vi "LA_data_decode_Rev01.vi"(10 "Data In":u8[](array[numeric])) -> (0 "Bytes Received":dbl, 1 "Time stamp":dbl, 2 "Data Bytes":dbl, 3 "RG15":u8[](array[numeric]), 4 "RG14":u8[](array[numeric]), 5 "All data":u8[](array[numeric]))   [LabVIEW 2012]
panel:
  out "Numeric 4":dbl
  out "Numeric 3":dbl
  out "Numeric 2":dbl
  out "Numeric":dbl
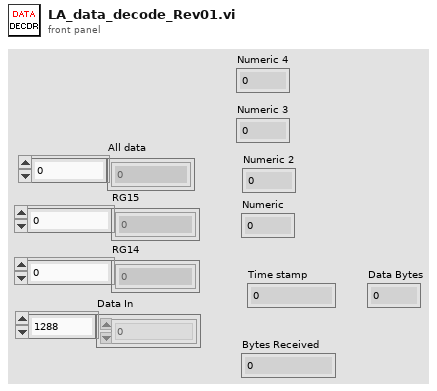
[diagram p1: front panel]
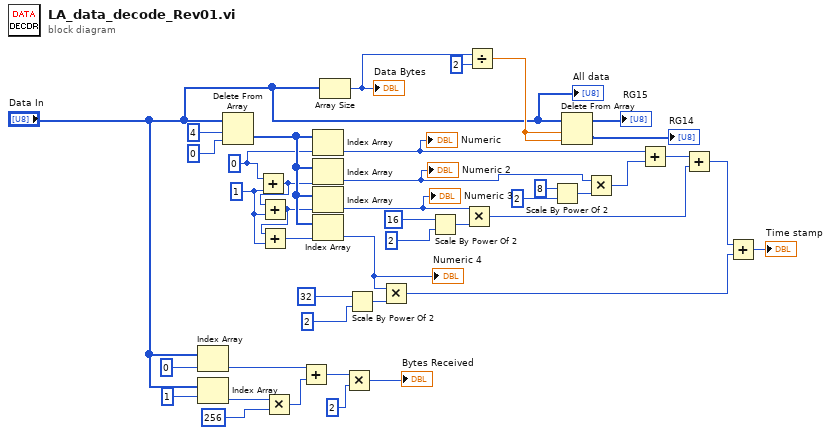
[diagram p0: block diagram]
diagram:
  w11 = 0
  w34 = 1
  n1 = Index Array(array="Data In", index=0) -> (element=w17:u8)
  n2 = Index Array(array="Data In", index=1) -> (element=w16:u8)
  n3 = Delete From Array(array="Data In", length=4, index=0) -> (deleted portion=w37:u8[])  [unwired: 1 out]
  n4 = Add(x=w11, y=w34) -> (x+y=w6:i32)
  n5 = Add(x=w6, y=w34) -> (x+y=w35:i32)
  n6 = Add(x=w35, y=w34) -> (x+y=w30:i32)
  n7 = Multiply(x=w16, y=256) -> (x*y=w39:i32)
  n8 = Add(x=w17, y=w39) -> (x+y=w10:i32)
  n9 = Index Array(array=w37, index=w11) -> (element=w15:u8)
  "Numeric" <- w15
  n10 = Index Array(array=w37, index=w6) -> (element=w14:u8)
  "Numeric 2" <- w14
  n11 = Index Array(array=w37, index=w35) -> (element=w13:u8)
  "Numeric 3" <- w13
  n12 = Index Array(array=w37, index=w30) -> (element=w12:u8)
  "Numeric 4" <- w12
  n13 = Array Size(array="Data In") -> (size(s)=w5:i32)
  "Data Bytes" <- w5
  n14 = Multiply(x=w10, y=2) -> (x*y=→"Bytes Received":i32)
  n15 = Scale By Power Of 2(n=32, x=2) -> (x*2^n=w33:i32)
  n16 = Multiply(x=w12, y=w33) -> (x*y=w19:i32)
  n17 = Scale By Power Of 2(n=16, x=2) -> (x*2^n=w29:i32)
  n18 = Multiply(x=w13, y=w29) -> (x*y=w21:i32)
  n19 = Divide(x=w5, y=2) -> (x/y=w3:dbl)
  n20 = Scale By Power Of 2(n=8, x=2) -> (x*2^n=w26:i32)
  n21 = Delete From Array(array="Data In", length=w3, index=w3) -> (deleted portion=→"RG14":u8[], array with subset deleted=→"RG15":u8[])
  n22 = Multiply(x=w14, y=w26) -> (x*y=w23:i32)
  n23 = Add(x=w15, y=w23) -> (x+y=w22:i32)
  n24 = Add(x=w22, y=w21) -> (x+y=w20:i32)
  n25 = Add(x=w20, y=w19) -> (x+y=→"Time stamp":i32)
  "All data" <- "Data In"
